vi "ConfigureSpectrum.vi"(7 "Resolution BW":dbl=520.0 caption="Resolution BW (MHz)", 8 "error in (no error)":errorcluster, 9 "center frequency":dbl=520.0 caption="Center Frequency (MHz)", 10 "span":dbl=1000.0 caption="Frequency span (MHz)", 11 "KeysightN9020B in":refnum<class "KeysightN9020B.lvclass">) -> (0 "error out":errorcluster, 3 "KeysightN9020B out":refnum<class "KeysightN9020B.lvclass">)   [LabVIEW 2023, in "KeysightN9020B.lvlib" / "KeysightN9020B.lvclass"]
uses:
  KeysightN9020B.lvclass
  KeysightN9020B.lvclass/KeysightN9020B.ctl
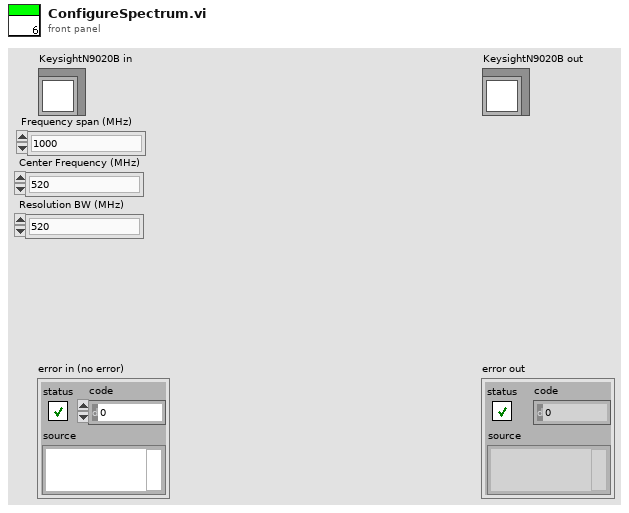
[diagram p1: front panel]
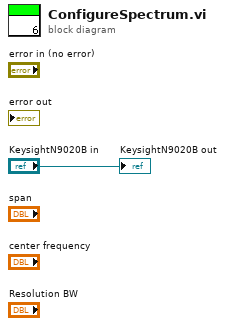
[diagram p0: block diagram]
diagram:
  "KeysightN9020B out" <- "KeysightN9020B in"
